vi "To Waveform.vi"(8 "error in (no error)":errorcluster, 11 "I32 Array in":refnum<class "I32 Array.lvclass">) -> (0 "error out":errorcluster, 1 "Success?":bool, 3 "Waveform Array":waveform(dbl)[](array[waveform]))   [LabVIEW 2020, in "Data.lvlib" / "I32 Array.lvclass"]
doc: "Interpret 'Data' as a Waveform Array. If impossible 'Success?' is set to FALSE"
uses:
  I32 Array.lvclass
  I32 Array.lvclass/I32 Array.ctl
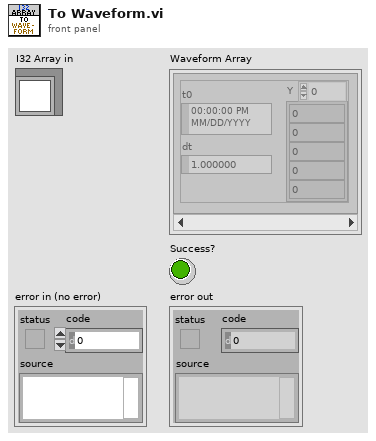
[diagram p1: front panel]
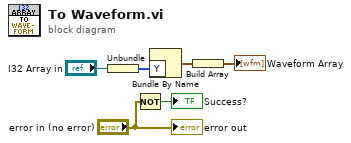
[diagram p0: block diagram]
diagram:
  n1 = Unbundle("I32 Array in") -> (w5:i32[])
  n2 = Not(x="error in (no error)") -> (.not. x?=→"Success?":bool)
  n3 = Bundle By Name("Y"=w5) -> (w6:waveform(i32))  [unwired: 1 in]
  n4 = Build Array(w6) -> (→"Waveform Array":waveform(i32)[])
  "error out" <- "error in (no error)"
